vi "Check Packets.vi"(10 "Right Packet":string, 11 "Left Packet":string) -> (2 "Terminated?":bool, 3 "Correct Order?":bool)   [LabVIEW 2021, in "d13.lvlib"]
uses:
  d13.lvlib
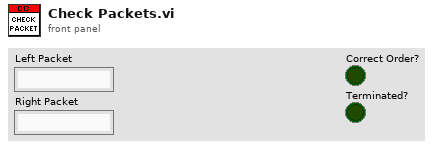
[diagram p1: front panel]
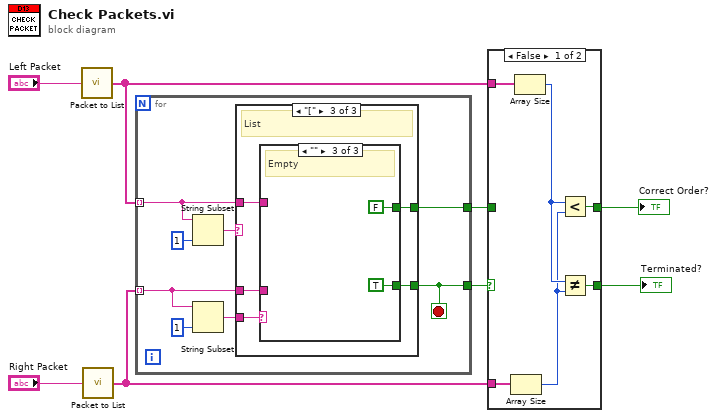
[diagram p0: block diagram]
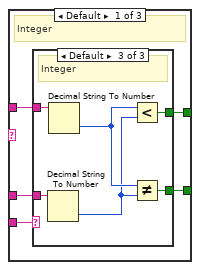
[diagram p3: hidden frame]
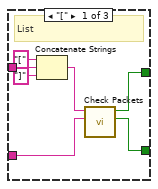
[diagram p4: hidden frame]
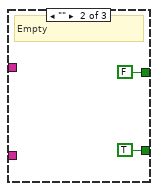
[diagram p5: hidden frame]
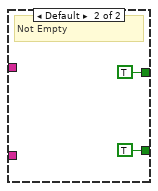
[diagram p7: hidden frame]
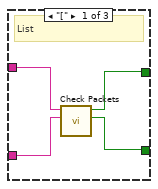
[diagram p8: hidden frame]
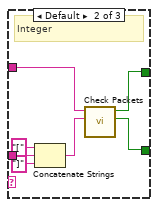
[diagram p9: hidden frame]
diagram:
  n1 = call "Packet to List.vi"("Packet"="Left Packet") -> ("List"=w2:string[])
  n2 = call "Packet to List.vi"("Packet"="Right Packet") -> ("List"=w1:string[])
  n3 = for {
    tunnel: w2 -> [w14] mode=indexing
    tunnel: w1 -> [w12] mode=indexing
    tunnel: [w10] -> w4
    tunnel: [w9] -> w6
    stop <- w9 stop-if-true
    n4 = String Subset(string=w14, length (rest)=1 ("length (rest)")) -> (substring=w15:string)  [unwired: 1 in]
    n5 = String Subset(string=w12, length (rest)=1 ("length (rest)")) -> (substring=w11:string)  [unwired: 1 in]
    n6 = case shown="\"[\"" w15 {
      tunnel: w14 -> [w20 w40 w47]
      tunnel: w12 -> [w19 w39 w46]
      tunnel: w11 -> [w21 w41 w48]
      tunnel: [w18 w38 w45] -> w9
      tunnel: [w17 w37 w44] -> w10
      frame Default {
        # "Integer"
        n7 = case shown="Default" w21 {
          tunnel: w20 -> [w28 _ w36]
          tunnel: w19 -> [w27 _ w34]
          tunnel: [w24 TRUE ("Terminated?") w35] -> w18
          tunnel: [w25 FALSE ("Correct Order?") w33] -> w17
          frame "[" {
            # "List"
            n8 = Concatenate Strings("[" ("string"), w28, "]" ("string")) -> (w26:string)
            n9 = call "Check Packets.vi"("Right Packet"=w27, "Left Packet"=w26) -> ("Terminated?"=w24:bool, "Correct Order?"=w25:bool)  [unwired: 8 in]
          }
          frame "" {
            # "Empty"
          }
          frame Default {
            # "Integer"
            n10 = Decimal String To Number(string=w34) -> (number=w31:i32)  [unwired: 2 in, 1 out]
            n11 = Decimal String To Number(string=w36) -> (number=w32:i32)  [unwired: 2 in, 1 out]
            n12 = Less?(x=w32, y=w31) -> (x < y?=w33:bool)
            n13 = Not Equal?(x=w32, y=w31) -> (x != y?=w35:bool)
          }
        }
      }
      frame "\u0000" {
        # "Empty"
        n14 = case shown="\"\"" w41 {
          tunnel: w40 -> [_ _]
          tunnel: w39 -> [_ _]
          tunnel: [_ TRUE ("Terminated?")] -> w38
          tunnel: [_ TRUE ("Correct Order?")] -> w37
          frame "" {
            # "Empty"
          }
          frame Default {
            # "Not Empty"
          }
        }
      }
      frame "[" {
        # "List"
        n15 = case shown="\"\"" w48 {
          tunnel: w47 -> [w49 w57 _]
          tunnel: w46 -> [w52 w53 _]
          tunnel: [w50 w58 TRUE ("Terminated?")] -> w45
          tunnel: [w51 w59 FALSE ("Correct Order?")] -> w44
          frame "[" {
            # "List"
            n16 = call "Check Packets.vi"("Right Packet"=w52, "Left Packet"=w49) -> ("Terminated?"=w50:bool, "Correct Order?"=w51:bool)  [unwired: 8 in]
          }
          frame Default {
            # "Integer"
            n17 = Concatenate Strings("[" ("string"), w53, "]" ("string")) -> (w54:string)
            n18 = call "Check Packets.vi"("Right Packet"=w54, "Left Packet"=w57) -> ("Terminated?"=w58:bool, "Correct Order?"=w59:bool)  [unwired: 8 in]
          }
          frame "" {
            # "Empty"
          }
        }
      }
    }
  }
  n19 = case shown="False" w6 {
    selector: w6 -> [_ w69]
    tunnel: [w65 w69] -> w5
    tunnel: w4 -> [_ w68]
    tunnel: [w64 w68] -> w3
    tunnel: w2 -> [w67 _]
    tunnel: w1 -> [w66 _]
    frame False {
      n20 = Array Size(array=w66) -> (size(s)=w62:i32)
      n21 = Array Size(array=w67) -> (size(s)=w63:i32)
      n22 = Less?(x=w63, y=w62) -> (x < y?=w64:bool)
      n23 = Not Equal?(x=w63, y=w62) -> (x != y?=w65:bool)
    }
    frame True {
    }
  }
  "Correct Order?" <- w3
  "Terminated?" <- w5
